vi "Curtin1_DeleteConfig.vi"(11 "Test Configuration":string) -> (3 "New File":string)   [LabVIEW 2022 SP3]
uses:
  Mic/Mic_Global.vi
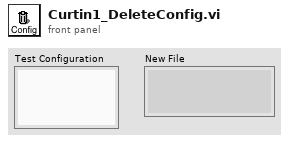
[diagram p1: front panel]
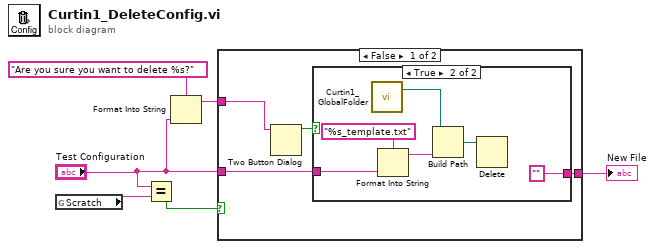
[diagram p0: block diagram]
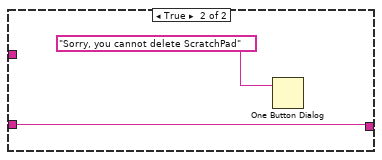
[diagram p3: hidden frame]
diagram:
  n1 = global read "Mic_Global.vi" "Scratch"() -> (w3:string)
  n2 = Equal?(x="Test Configuration", y=w3) -> (x = y?=w1:bool)
  n3 = Format Into String(format string="Are you sure you want to delete %s?" ("message"), "Test Configuration") -> (resulting string=w4:string)  [unwired: 2 in, 1 out]
  n4 = case shown="False" w1 {
    tunnel: [w9 w19] -> w6
    tunnel: "Test Configuration" -> [w10 w19]
    tunnel: w4 -> [w7 _]
    frame False {
      n5 = Two Button Dialog(message=w7) -> (T button?=w8:bool)  [unwired: 2 in]
      n6 = case shown="True" w8 {
        tunnel: w10 -> [w11 w16]
        tunnel: [w11 "" ("Test Configuration")] -> w9
        frame False {
        }
        frame True {
          n7 = call "Curtin1_GlobalFolder.vi"() -> ("LabVIEW Data Path"=w15:path)  [unwired: 1 in, 1 out]
          n8 = Format Into String(format string="%s_template.txt" ("pattern"), w16) -> (resulting string=w14:string)  [unwired: 2 in, 1 out]
          n9 = Build Path(base path=w15, name or relative path=w14) -> (appended path=w13:path)
          n10 = Delete(path (use dialog)=w13) -> ()  [unwired: 4 in, 3 out]
        }
      }
    }
    frame True {
      n11 = One Button Dialog(message="Sorry, you cannot delete ScratchPad") -> ()  [unwired: 1 in, 1 out]
    }
  }
  "New File" <- w6
